vi "Read Address.vi"(11 "Notifier Transport in":refnum<class "Notifier Transport.lvclass">) -> (2 "Address":refnum<data-value>)   [LabVIEW 2025, in "jettl.lvlib" / "Notifier Transport.lvlib" / "Notifier Transport.lvclass"]
uses:
  Notifier Transport.lvclass
  Notifier Transport.lvclass/Notifier Transport.ctl
  Msg/Msg.lvclass
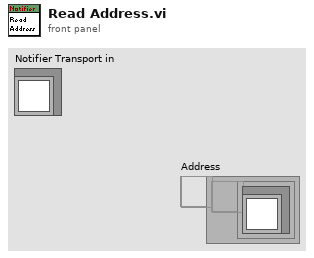
[diagram p1: front panel]
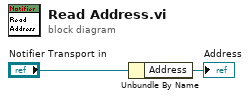
[diagram p0: block diagram]
diagram:
  n1 = Unbundle By Name("Notifier Transport in") -> ("Address"=→"Address":refnum<data-value>)
